vi "Do.vi"(7 "Topic Actor in":refnum<class "Topic Actor.lvclass">, 8 "error in (no error)":errorcluster, 11 "Topic Actor Command in":refnum<class "Topic Actor Subscribe Command.lvclass">) -> (0 "error out":errorcluster, 3 "Topic Actor Command out":refnum<class "Topic Actor Subscribe Command.lvclass">, 5 "Topic Actor out":refnum<class "Topic Actor.lvclass">)   [LabVIEW 2016, in "Stream Mediator.lvlib" / "Topic Actor Subscribe Command.lvclass"]
doc: "--\nCopyright © 2017 Composed SystemsI All rights reserved.\n\nAuthor: Jon McBee <jon.mcbee@composed.io>\n\nThis library is provided \"AS IS\" ,WITHOUT WARRANTIES OR\nCONDITIONS OF ANY KIND, either express or implied.\n\nComposed Systems -- composed.io\n\nStream 0.0.1.1\nJon McBee - Composed Systems\nCopyright (c) 2017, Composed Systems"
uses:
  <userlib>/Composed Systems/Stream/Mediator/Classes/Topic Actor Subscribe Command/Topic Actor Subscribe Command.lvclass
  <userlib>/Composed Systems/Stream/Mediator/Classes/Topic Actor/Topic Actor.lvclass
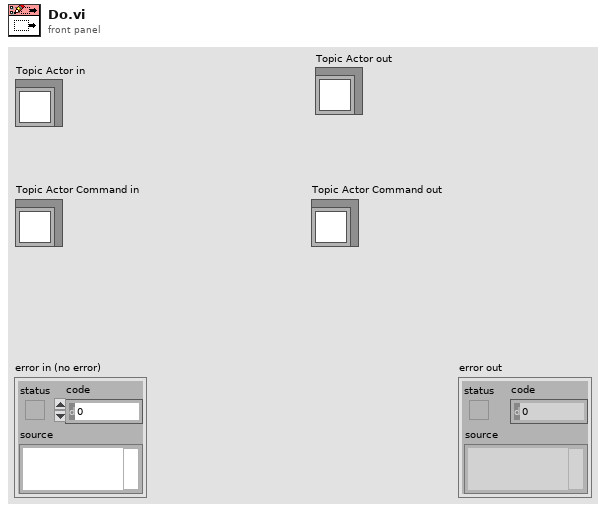
[diagram p1: front panel]
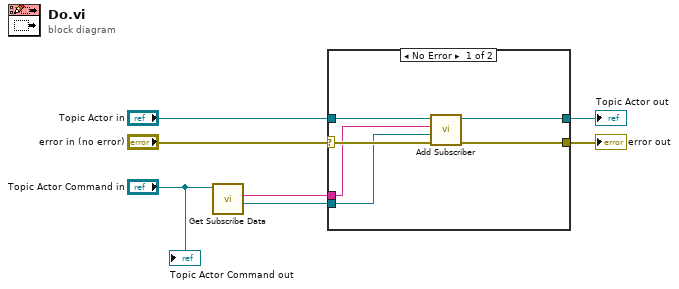
[diagram p0: block diagram]
diagram:
  n1 = call <userlib>:"Get Subscribe Data.vi"("Topic Actor Subscribe Command in"="Topic Actor Command in") -> ("Message Transport Interface"=w2:refnum<class "Message Transport Interface.lvclass">, "Subscriber Name"=w3:string)  [unwired: 7 in, 2 out]
  n2 = case shown="No Error" "error in (no error)" {
    selector: "error in (no error)" -> [w13 w14]
    tunnel: [w10 _] -> w6
    tunnel: "Topic Actor in" -> [w11 _]
    tunnel: w3 -> [w9 _]
    tunnel: w2 -> [w8 _]
    tunnel: [w12 w14] -> w1
    frame No Error {
      n3 = call <userlib>:"Add Subscriber.vi"("error in (no error)"=w13, "Message Transport Interface"=w8, "Topic Name"=w9, "Topic Actor in"=w11) -> ("error out"=w12:errorcluster, "Topic Actor out"=w10:refnum<class "Topic Actor.lvclass">)  [unwired: 6 in]
    }
    frame Error {
    }
  }
  "error out" <- w1
  "Topic Actor out" <- w6
  "Topic Actor Command out" <- "Topic Actor Command in"
